vi "configure.vi"(8 "error in (no error)":errorcluster, 11 "ScanModeMG090624Camera in":refnum<class "ImagingModeMG090624Camera.lvclass">) -> (0 "error out":errorcluster, 3 "ScanModeMG090624Camera out":refnum<class "ImagingModeMG090624Camera.lvclass">)   [LabVIEW 2010, in "ImagingModeMG090624Camera.lvclass"]
doc: "The dynamic dispatch version of this VI loads and displays the configuration file associated with the plug-in object. The user modify and save the configuration data."
uses:
  ImagingModeMG090624Camera.lvclass
  ImagingModeDL090923Scaffold/ImagingModeDL090923Scaffold/configuration_visibility_cluster.ctl
  ImagingModeDL090923Scaffold/ImagingModeDL090923Scaffold/component_configuration_visibility_cluster.ctl
  ImagingModeDL090923Scaffold/ImagingModeDL090923Scaffold/ImagingModeDL090923Scaffold.lvclass
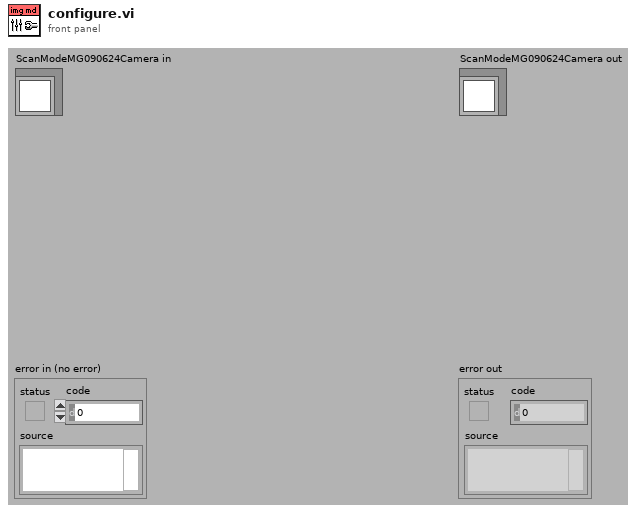
[diagram p1: front panel]
types:
  T1 = typedef "ImagingModeDL090923Scaffold.lvclass/configuration_visibility_cluster.ctl" = cluster{"Instrument":T2, "Trajectory":T2, "ScanHead":T2, "DAQ":T2, "ImageAssembler":T2, "DataCollection":T2, "Display":T2, "Analyser":T2, "Stimulator":T2, "enable Trajectory-to-ImageAssembler adapter":bool}
  T2 = typedef "ImagingModeDL090923Scaffold.lvclass/component_configuration_visibility_cluster.ctl" = cluster{"enable":bool, "enable adapter":bool}
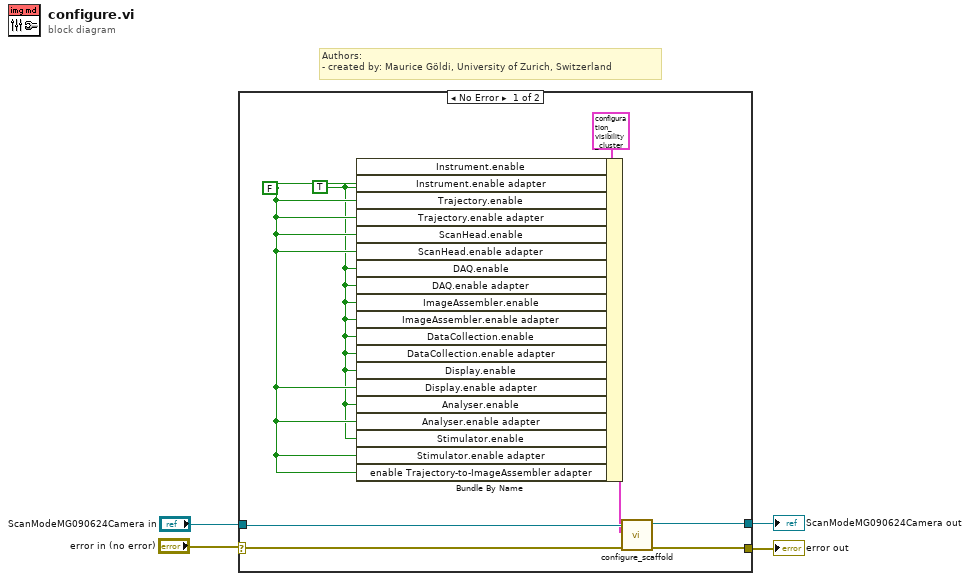
[diagram p0: block diagram]
diagram:
  # "Authors: \n- created by: Maurice Göldi, University of Zurich, Switzerland"
  n1 = case shown="No Error" "error in (no error)" {
    selector: "error in (no error)" -> [w12 w14]
    tunnel: [w8 w14] -> w3
    tunnel: "ScanModeMG090624Camera in" -> [w11 w13]
    tunnel: [w7 w13] -> w1
    frame No Error {
      w6 = FALSE
      w5 = TRUE
      n2 = Bundle By Name(cluster=T1 {"Instrument"={"enable"=FALSE, "enable adapter"=FALSE}, "Trajectory"={"enable"=FALSE, "enable adapter"=FALSE}, "ScanHead"={"enable"=FALSE, "enable adapter"=FALSE}, "DAQ"={"enable"=FALSE, "enable adapter"=FALSE}, "ImageAssembler"={"enable"=FALSE, "enable adapter"=FALSE}, "DataCollection"={"enable"=FALSE, "enable adapter"=FALSE}, "Display"={"enable"=FALSE, "enable adapter"=FALSE}, "Analyser"={"enable"=FALSE, "enable adapter"=FALSE}, "Stimulator"={"enable"=FALSE, "enable adapter"=FALSE}, "enable Trajectory-to-ImageAssembler adapter"=FALSE} ("visibilities"), "Instrument.enable"=w5, "Instrument.enable adapter"=w6, "Trajectory.enable"=w6, "Trajectory.enable adapter"=w6, "ScanHead.enable"=w6, "ScanHead.enable adapter"=w6, "DAQ.enable"=w5, "DAQ.enable adapter"=w5, "ImageAssembler.enable"=w5, "ImageAssembler.enable adapter"=w5, "DataCollection.enable"=w5, "DataCollection.enable adapter"=w5, "Display.enable"=w5, "Display.enable adapter"=w6, "Analyser.enable"=w5, "Analyser.enable adapter"=w6, "Stimulator.enable"=w5, "Stimulator.enable adapter"=w6, "enable Trajectory-to-ImageAssembler adapter"=w6) -> (w10:T1)
      n3 = call-dynamic "configure_scaffold.vi"("error in (no error)"=w12, "visibilities"=w10, "ScanModeDL090923Scaffold in"=w11) -> ("error out"=w8:errorcluster, "ScanModeDL090923Scaffold out"=w7:refnum<class "ImagingModeMG090624Camera.lvclass">)  [unwired: 7 in]
    }
    frame Error {
    }
  }
  "error out" <- w3
  "ScanModeMG090624Camera out" <- w1
